vi "Sub Panel.vi"   [LabVIEW 2019, in "ModuleD.lvclass"]
uses:
  ModuleD.lvclass
  ModuleC/ModuleC.lvlib
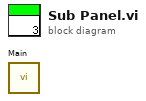
[diagram p0: block diagram]
diagram:
  n1 = call "Main.vi"() -> ()  [unwired: 12 in]
